vi "HV_ISet_Single.vi"(9 "Current":string, 10 "Channel":string) -> (2 "Output":string)   [LabVIEW 2019]
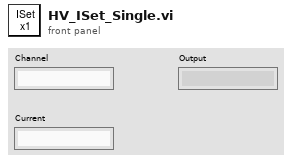
[diagram p1: front panel]
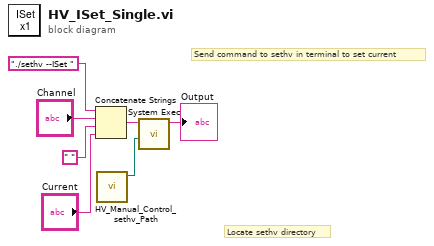
[diagram p0: block diagram]
diagram:
  # "Locate sethv directory"
  # "Send command to sethv in terminal to set current"
  n1 = Concatenate Strings("./sethv --ISet ", "Channel", " ", "Current") -> (w3:string)
  n2 = call "HV_Manual_Control_sethv_Path.vi"() -> ("sethv filepath"=w1:path)  [unwired: 11 in]
  n3 = call <vilib>:"System Exec.vi"("working directory"=w1, "command line"=w3) -> ("standard output"=→"Output":string)  [unwired: 6 in, 3 out]
